vi "HTSuperProReadAnalog.vi"(0 "Analog Port":u8(ring) items=["A0", "A1", "A2", "A3"], 3 "NXT":T1={"error"={"status"=FALSE, "code"=0, "source"=""}, "address"="", "NXT #"=-1, "Show Error"=TRUE, "Connection"=4} {"Connection" items=["USB", "Bluetooth", "USB then Bluetooth", "Last Connection", "Preference"]}, 4 "Port":T2 items=["Port 1", "Port 2", "Port 3", "Port 4"]) -> (2 "Analog Value":i16, 5 "NXT":T1={"error"={"status"=FALSE, "code"=0, "source"=""}, "address"="", "NXT #"=-1, "Show Error"=TRUE, "Connection"=4} {"Connection" items=["USB", "Bluetooth", "USB then Bluetooth", "Last Connection", "Preference"]})   [LabVIEW 2009]
doc: "HiTechnic SuperPro - Read Analog\n\n<B>Inputs\nPort </B> is the port connected to the sensor. Port 1 is the default, but Port 2, Port 3, or Port 4 can also be selected.\n<B>NXT </B> connects to NXT terminal of previous VI to establish the flow of the program.\n<B>Analog Port</B> either A0, A1, A2, or A3\n\n<B>Outputs\nNXT </B> wires to NXT terminal of next VI to establish the flow of the program.\n<B>Analog Value </B> analog value form specified analog port. Value range of 0-1023 corresponds to 0-3.3v"
uses:
  <vilib>/NXT/Block Support/NXT_InputPort.ctl
  <vilib>/NXT/Subs/LVHSConnector.ctl
  <vilib>/NXT/Block Support/HWPage.SensorType.ctl
  <vilib>/NXT/Block Support/HWPage.SensorMode.ctl
panel:
  # "HiTechnic SuperPro Prototype board VI\nRead Analog\n\nRead one of the four analog ports on the SuperPro.  The voltage at the analog port is a 10 bit value with a range of 0 to 1023 corresponding to 0-3.3v.\n\n(c) HiTechnic 2011"
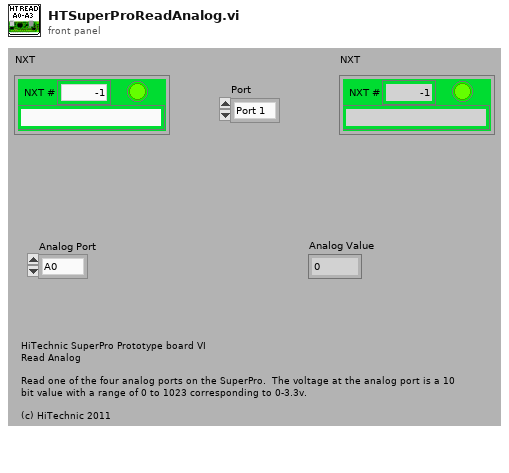
[diagram p1: front panel]
types:
  T1 = typedef "LVHSConnector.ctl" = cluster{"error":errorcluster, "address":string, "NXT #":i32, "Show Error":bool, "Connection":u16}
  T2 = typedef "NXT_InputPort.ctl" = u8
  T3 = typedef "HWPage.SensorType.ctl" = u8
  T4 = typedef "HWPage.SensorMode.ctl" = u8
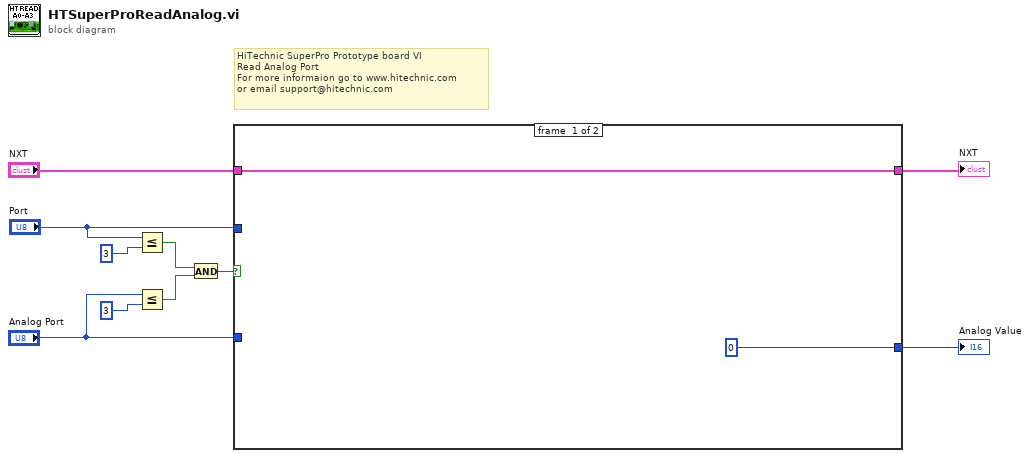
[diagram p0: block diagram]
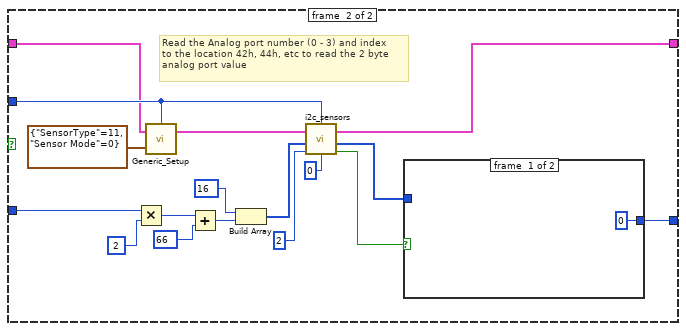
[diagram p2: hidden frame]
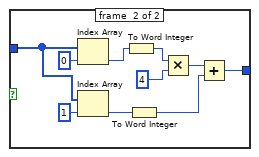
[diagram p3: hidden frame]
diagram:
  # "HiTechnic SuperPro Prototype board VI\nRead Analog Port\nFor more informaion go to www.hitechnic.com\nor email support@hitechnic.com"
  n1 = Less Or Equal?(x="Port", y=u8 3) -> (x <= y?=w4:bool)
  n2 = Less Or Equal?(x="Analog Port", y=u8 3) -> (x <= y?=w5:bool)
  n3 = And(x=w4, y=w5) -> (x .and. y?=w3:bool)
  n4 = case shown="True" w3 {
    tunnel: "Port" -> [_ w27]
    tunnel: "Analog Port" -> [_ w29]
    tunnel: "NXT" -> [w11 w26]
    tunnel: [w11 w24] -> w8
    tunnel: [i16 0 w23] -> w7
    frame #0 {
    }
    frame #1 {
      # "Read the Analog port number (0 - 3) and index\nto the location 42h, 44h, etc to read the 2 byte\nanalog port value"
      n5 = Multiply(x=w29, y=u8 2) -> (x*y=w21:u8)
      n6 = call <vilib>:"Generic_Setup.vi"("Sensor Setup"=cluster{"SensorType":T3, "Sensor Mode":T4} {"SensorType"=11, "Sensor Mode"=0}, "NXT"=w26, "Port"=w27) -> ("NXT"=w25:T1)  [unwired: 1 out]
      n7 = Add(x=w21, y=u8 66) -> (x+y=w18:u8)
      n8 = Build Array(u8 16, w18) -> (w17:u8[])
      n9 = call <vilib>:"i2c_sensors.vi"("Return Length"=u8 2, "Bytes to Write"=w17, "Wait (msec)"=u32 0, "NXT"=w25, "Port"=w27) -> ("Success?"=w15:bool, "Bytes read"=w14:u8[], "NXT"=w24:T1)
      n10 = case shown="True" w15 {
        tunnel: w14 -> [_ w36]
        tunnel: [i16 0 w31] -> w23
        frame #0 {
        }
        frame #1 {
          n11 = Index Array(array=w36, index=0) -> (element=w35:u8)
          n12 = Index Array(array=w36, index=1) -> (element=w33:u8)
          n13 = To Word Integer(number=w35) -> (16bit integer=w34:i16)
          n14 = To Word Integer(number=w33) -> (16bit integer=w32:i16)
          n15 = Multiply(x=w34, y=i16 4) -> (x*y=w39:i16)
          n16 = Add(x=w39, y=w32) -> (x+y=w31:i16)
        }
      }
    }
  }
  "NXT" <- w8
  "Analog Value" <- w7
